vi "myRIO-1900 Quadrotor Sensor FPGA.vi"() -> ()   [LabVIEW 2013]
uses:
  <vilib>/Platform/TimedLoop/XDataNode/timing_clust.ctl
  <vilib>/Platform/TimedLoop/XDataNode/nitl_modes.ctl
  <vilib>/Platform/TimedLoop/XDataNode/wakeup.ctl
  <vilib>/IEDriver/SPIandI2C/FPGA/Private/Initialize Port (I2C).vi
  <vilib>/IEDriver/SPIandI2C/FPGA/Private/IP Port (I2C).vi
  <vilib>/rvi/DataTransferAndStorage/Container/Common/niFpgaContainerGetUniqueNameForEmu.vi
  <vilib>/rvi/DataTransferAndStorage/Container/Common/niFpgaContainerSetEmuInfo.vi
  <vilib>/rvi/eio/common/nirviEmuReportErrorAndStop.vi
  <vilib>/rvi/Emulation/niFpgaSctlEmulationGetInTimedLoop.vi
  <vilib>/rvi/Emulation/niFpgaEmulationReportErrorSimple.vi
  <vilib>/rvi/Emulation/niFpgaGetClockAttributes.vi
  <vilib>/rvi/Emulation/niFpgaCriticalErrorInLSC.vi
  <vilib>/rvi/DataTransferAndStorage/Container/Common/niFpgaContainerExecOnDevCompGetState.vi
  <vilib>/rvi/FIFO/Fifo_Resource/nirvififoEmulationReadFpgaImpl.vi
  <vilib>/rvi/interface/RandomDataEmulation/nirviRandomDataFPGAFIFO.vi
  <vilib>/rvi/interface/RandomDataEmulation/niFpgaRandomDataHandleErrors.vi
  <vilib>/rvi/Memory/Memory_Emulation/nirvimemoryFastEmulationFpgaImpl.vi
  <instcachedir>/0/nirvimemoryFastEmulationFpgaImpl_5FBAB50466BC4C939F684F8805638BFC.lvgen/nirvimemoryFastEmulationFpgaImpl_5FBAB50466BC4C939F684F8805638BFC_005.vi
  <vilib>/rvi/Memory/Memory_Emulation/niFpgaMemoryEmulationCacheClearOnFirstRun.vi
  <vilib>/rvi/Memory/Memory_Emulation/nirvimemoryEmulationManagerCache_MakeExclusive.vi
  <vilib>/rvi/Memory/Memory_Emulation/niFpgaMemoryEmulationValidateCache.vi
  <vilib>/rvi/Memory/Memory_Emulation/nirvimemoryEmulationManagerCache_ReleaseExclusive.vi
  <vilib>/rvi/Memory/Memory_Emulation/nirvimemoryEmulationManagerCache_InsertValue.vi
  <vilib>/Utility/error.llb/Clear Errors.vi
  <vilib>/rvi/Memory/Memory_Emulation/nirvimemoryEmulationManagerCache_GetValue.vi
  <vilib>/rvi/Emulation/niFpgaProcessEmulError.vi
  <vilib>/IEDriver/SPIandI2C/FPGA/Private/Configure Port (I2C).vi
  <vilib>/IEDriver/SPIandI2C/FPGA/Private/Arm Port (I2C).vi
  <vilib>/IEDriver/SPIandI2C/FPGA/Private/Read Port (I2C).vi
  <vilib>/IEDriver/SPIandI2C/FPGA/Private/Write Port (I2C).vi
  <vilib>/rvi/FIFO/Fifo_Resource/nirvififoEmulationWriteFpgaImpl.vi
  <vilib>/rvi/Memory/Memory_Emulation/nirvimemoryEmulationManagerCache_SetValue.vi
  <vilib>/rvi/Emulation/niFpgaSctlEmulationResourceMgr.vi
  <vilib>/Platform/TimedLoop/XDataNode/XDataNode.xnode
  <vilib>/rvi/LocalResourceManager/LocalResourceManager.xnode
  <vilib>/rvi/DataTransferAndStorage/Container/XNode/niFpgaContainer.xnode
  <vilib>/rvi/FIFO/Fifo_Resource/niFpgaFifoEmulationRefIn.vi
  <vilib>/rvi/Memory/Memory_Emulation/niFpgaMemoryEmulationRefIn.vi
  <vilib>/IEDriver/SPIandI2C/FPGA/Library/IP SPI&I2C.lvlib
  <vilib>/Platform/TimedLoop/XDataNode/XDNodeRunTimeDep.lvlib
panel:
  in  "DataAva":bool
  out "GYR_Z":i16
  out "GYR_Y":i16
  out "GYR_X":i16
  out "TEMP":i16
  out "ACC_Z":i16
  out "ACC_Y":i16
  out "ACC_X":i16
  in  "SampleRate_Divider":u32=20000
  in  "WriteData":u8 format="0x%x"
  out "ReadData":u8 format="0x%x"
  in  "CMDParameters":T1
  in  "IICParameters":T2={"Address Type (7-bit)"=enum."7-bit", "IICSlaveAddress"=25, "I2C Parameters"={"Clock Divider"=0}} {"IICSlaveAddress" format="0x%x"}
  in  "ProtocolControl":T3(ring)
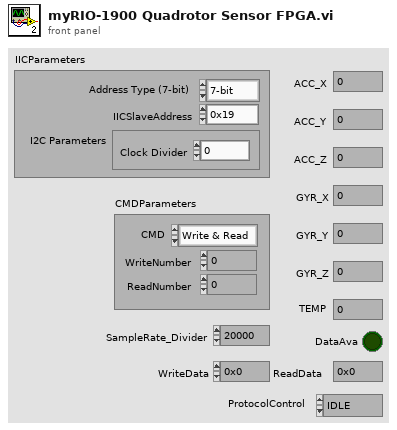
[diagram p1: front panel]
types:
  T1 = cluster{"WriteNumber":u8, "ReadNumber":u8, "CMD":enum8{"Write & Read", "Write", "Read"}}
  T2 = cluster{"Address Type (7-bit)":enum16{"7-bit", "10-bit"}, "IICSlaveAddress":u16, "I2C Parameters":cluster{"Clock Divider":u32}}
  T3 = enum8{"IDLE", "SetIDLE", "Config", "Arm", "Read", "Write", "AutoRead"}
  T4 = cluster{"MPU6050FIFO":refnum<k21>, "MPU6050FIFOAvailable":refnum<k21>}
  T5 = typedef "IP SPI&I2C.lvlib/Private Data (I2C).ctl" = cluster{"Arm Trigger":refnum<k21>, "API to IP Data":refnum<k21>, "IP to API Data":refnum<k21>, "Configuration Register":refnum<k21>, "Configuration Lock":refnum<k21>}
  T6 = typedef "XDNodeRunTimeDep.lvlib/timing_clust.ctl" = cluster{"Expected End [f-1]":u64, "Actual End [f-1]":u64, "Finished Late? [f-1]":bool, "Expected End [i-1]":u64, "Actual End [i-1]":u64, "Finished Late? [i-1]":bool, "Expected Start [i]":u64, "Actual Start [i]":u64, "Expected Start [f]":u64, "Actual Start [f]":u64, "Source Name":string, "Structure Name":string, "Period":i64, "Deadline":i64, "Offset":i64, "Start":i64, "Priority":i32, "Timeout":i32, "Mode":T7, "Wakeup Reason":T8, "Error":errorcluster, "Source Type":string, "Secondary Source Type":string, "Global End Time":u64, "Global Start Time":u64, "Frame Duration":u64, "Iteration Duration":u64, "Assigned CPU":i32, "I/O Scan Engine Mode":u32}
  T7 = typedef "XDNodeRunTimeDep.lvlib/nitl_modes.ctl" = enum32{"No Change", "Process missed periods, maintain original phase", "Discard missed periods, maintain original phase", "Process missed periods, ignore original phase", "Discard missed periods, ignore original phase"}
  T8 = typedef "XDNodeRunTimeDep.lvlib/wakeup.ctl" = enum32{"Normal", "Aborted", "Asynchronous wakeup", "Timing source error", "Timed loop error", "Timeout"}
  T9 = cluster{"NextState":enum16{"Configure", "WriteAddr", "Arm", "Read", "Wait", "Stop"}, "ReadCount":u8, "WaitCounter":u32}
  T10 = enum16{"Configure", "WriteAddr", "Arm", "Read", "Wait", "Stop"}
  T11 = cluster{"NextState":enum8{"IDLE", "ReadData", "Update"}, "ReadCounter":u8, "HighByte":u8}
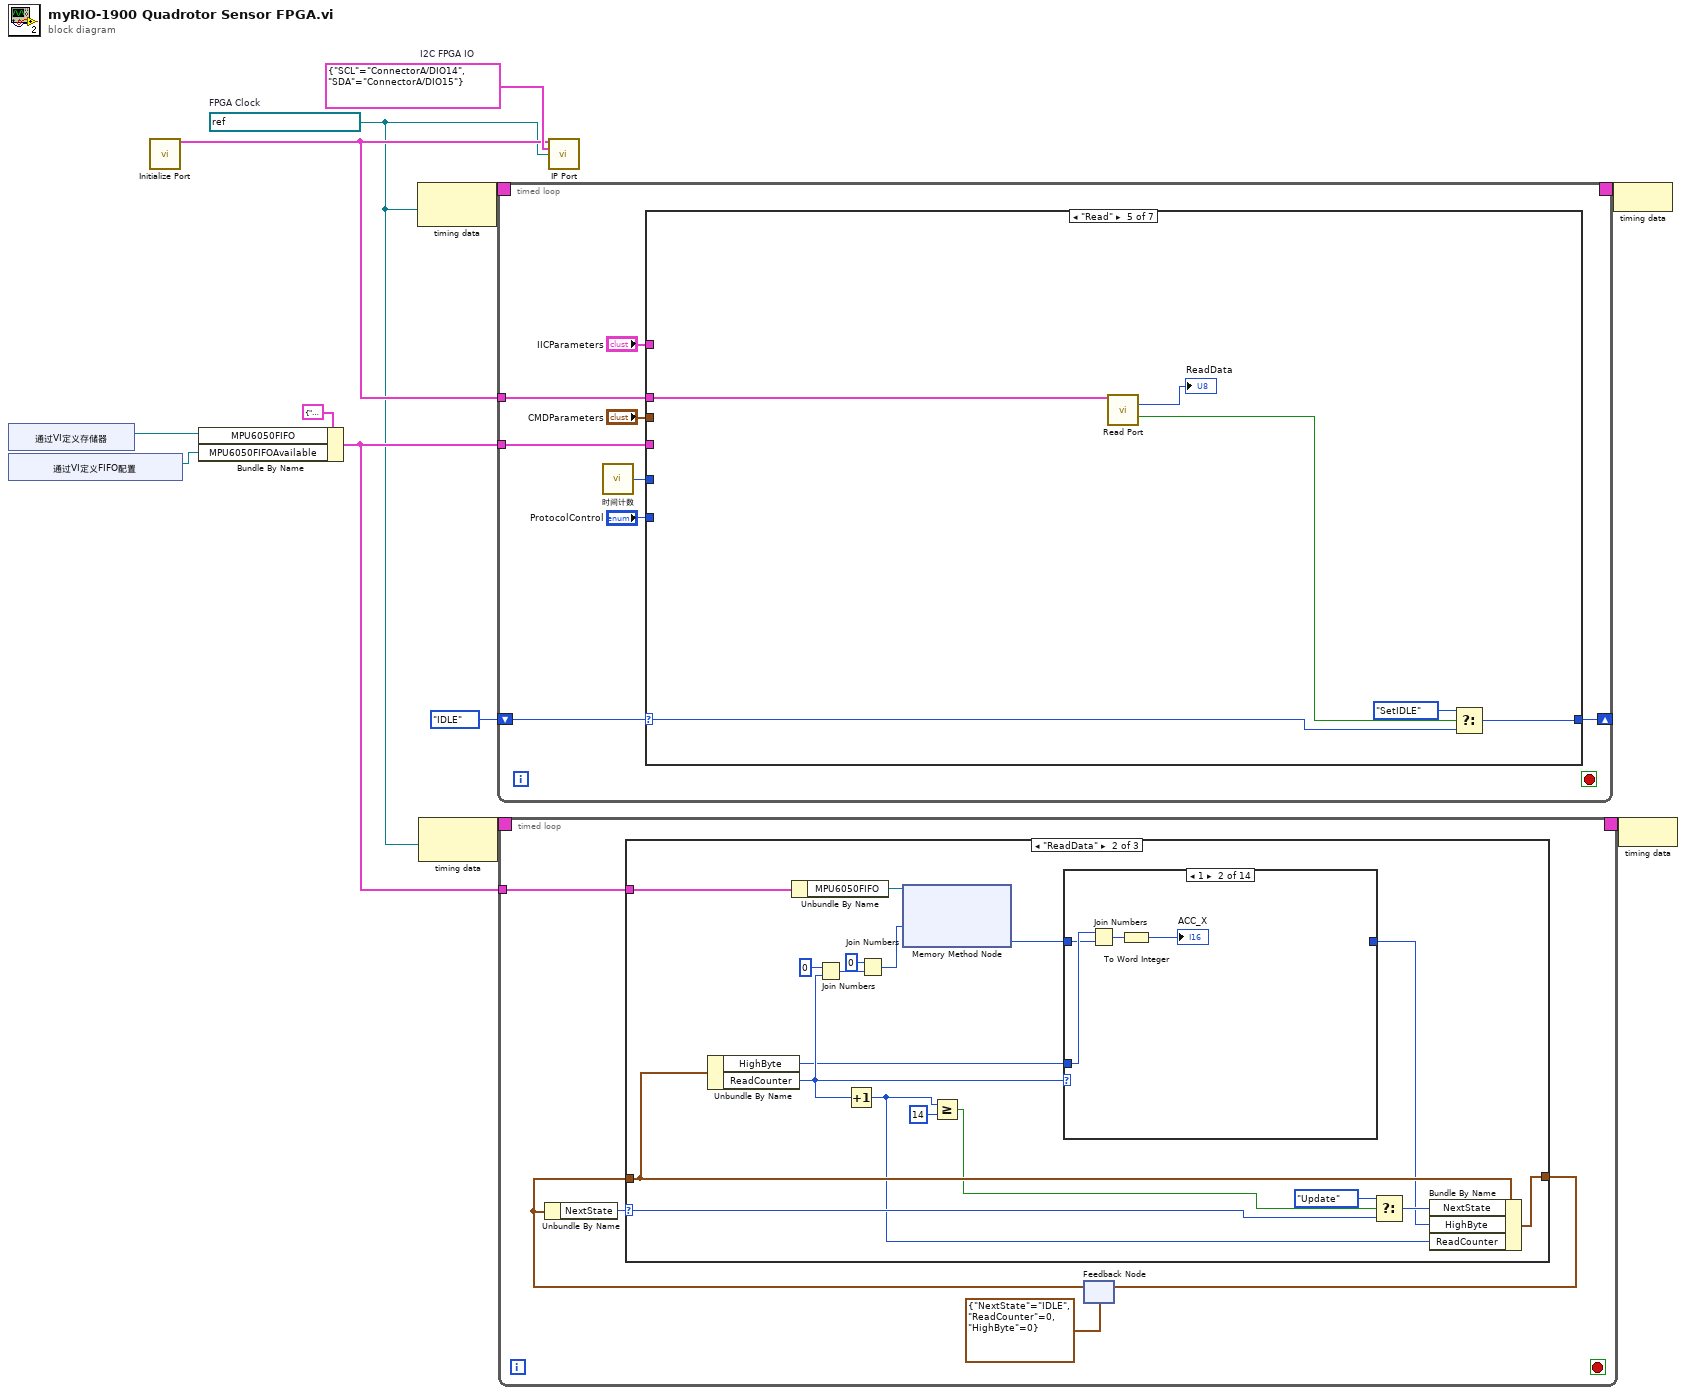
[diagram p0: block diagram]
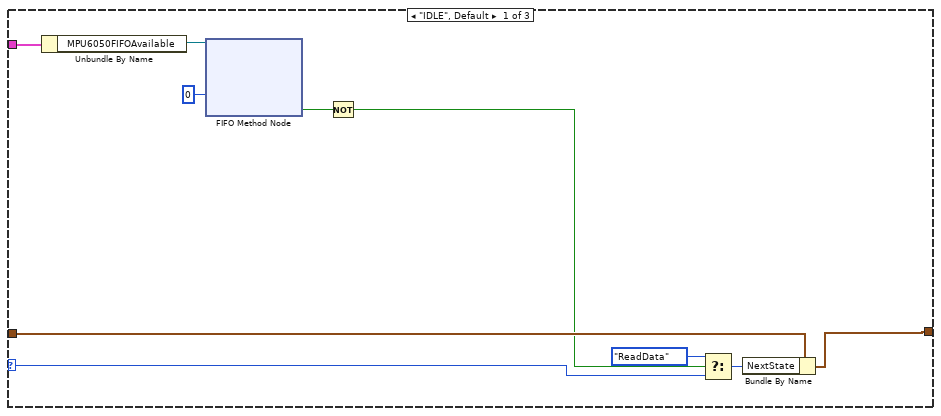
[diagram p2: hidden frame]
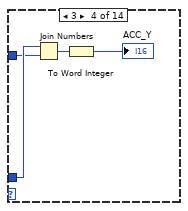
[diagram p5: hidden frame]
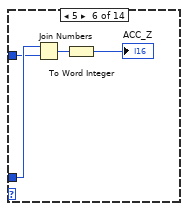
[diagram p7: hidden frame]
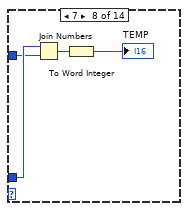
[diagram p9: hidden frame]
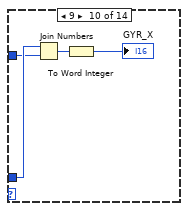
[diagram p11: hidden frame]
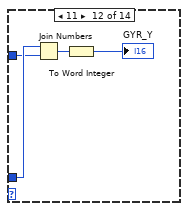
[diagram p13: hidden frame]
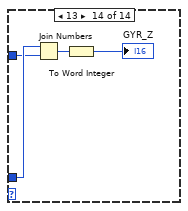
[diagram p15: hidden frame]
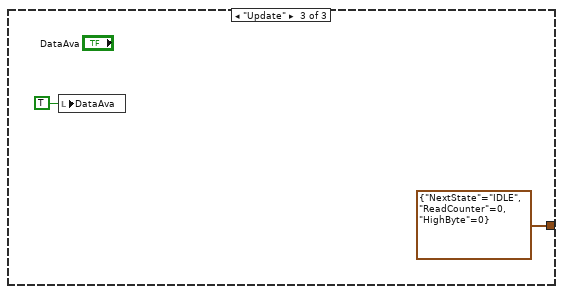
[diagram p16: hidden frame]
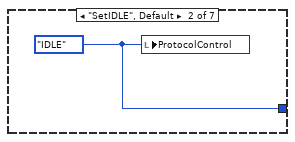
[diagram p18: hidden frame]
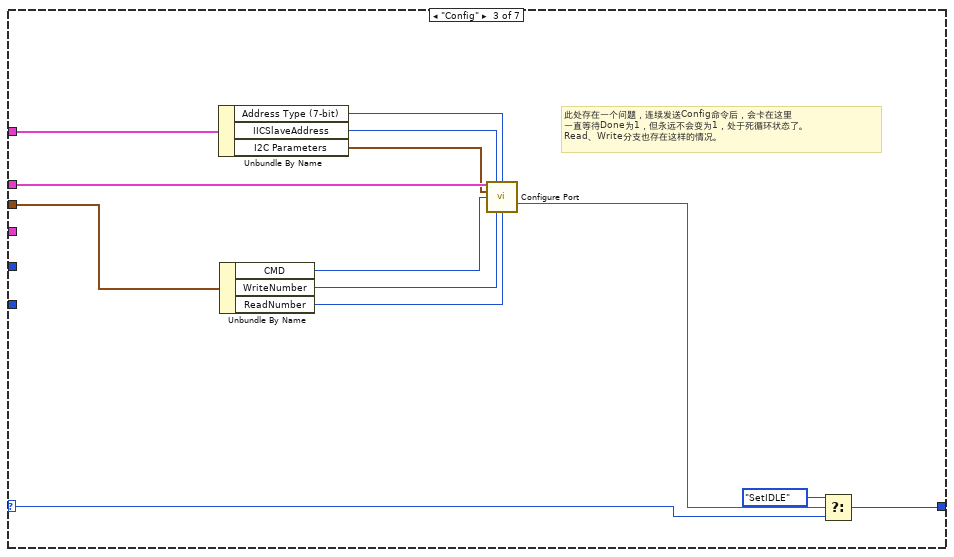
[diagram p19: hidden frame]
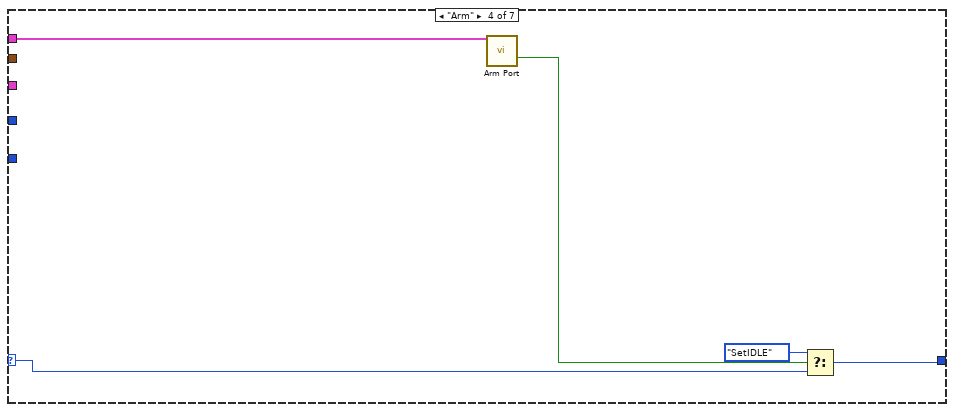
[diagram p20: hidden frame]
diagram:
  w1 = refnum<k21> "40 MHz Onboard Clock"  # FPGA Clock
  w8 = cluster{"SCL":refnum<k21>, "SDA":refnum<k21>} {"SCL"="ConnectorA/DIO14", "SDA"="ConnectorA/DIO15"}  # I2C FPGA IO
  n1 = xnode "通过VI定义存储器"() -> ("存储器输出"=w4:refnum<k21>)
  n2 = xnode "通过VI定义FIFO配置"() -> ("FIFO输出"=w3:refnum<k21>)
  n3 = call-poly <vilib>:"Initialize Port.vi"() -> ("Private Data Out"=w7:T5)  [unwired: 14 in, 1 out]
  n4 = Bundle By Name(cluster=T4 {"MPU6050FIFO"="", "MPU6050FIFOAvailable"=""}, "MPU6050FIFO"=w4, "MPU6050FIFOAvailable"=w3) -> (w2:T4)
  n5 = node-c288(w1) -> (w12:T6)
  n6 = node-c288(w1) -> (w10:T6)
  n7 = timed-loop {
    tunnel: w7 -> [w18]
    shift-right: [w15] -> _
    shift-left: T3."IDLE" ("ProtocolControl") -> [w20]
    timing: w12 -> [_]
    timing-out: [_] -> w11
    tunnel: w2 -> [w13]
    stop <- _ stop-if-true
    n8 = call "时间计数"() -> ("Tick Count(Ticks)"=w14:u32)
    n9 = case shown="\"Read\"" w20 {
      selector: w20 -> [_ _ w35 w38 w45 w50 w63]
      tunnel: "CMDParameters" -> [_ _ w28 _ _ _ _]
      tunnel: w18 -> [_ _ w34 w40 w46 w52 w59]
      tunnel: "IICParameters" -> [_ _ w32 _ _ _ w58]
      tunnel: "ProtocolControl" -> [w21 _ _ _ _ _ w57]
      tunnel: [w21 w22 w24 w37 w42 w48 w64] -> w15
      tunnel: w14 -> [_ _ _ _ _ _ w55]
      tunnel: w13 -> [_ _ _ _ _ _ w54]
      frame "IDLE" {
      }
      frame "SetIDLE", Default {
        w22 = T3."IDLE" ("ProtocolControl")
        n10 = local write "ProtocolControl"(w22) -> ()
      }
      frame "Config" {
        # "此处存在一个问题，连续发送Config命令后，会卡在这里\n一直等待Done为1，但永远不会变为1，处于死循环状态了。\nRead、Write分支也存在这样的情况。"
        n11 = Unbundle By Name(w32) -> ("Address Type (7-bit)"=w31:enum16{"7-bit", "10-bit"}, "IICSlaveAddress"=w30:u16, "I2C Parameters"=w29:cluster{"Clock Divider":u32})
        n12 = Unbundle By Name(w28) -> ("CMD"=w27:enum8{"Write & Read", "Write", "Read"}, "WriteNumber"=w26:u8, "ReadNumber"=w25:u8)
        n13 = call-poly <vilib>:"Configure Port.vi"("Private Data In"=w34, "Address"=w30, "Address Type (7-bit)"=w31, "I2C Parameters"=w29, "Command (Write & Read)"=w27, "Number of Bytes to Write"=w26, "Number of Bytes to Read"=w25) -> ("Done"=w33:bool)  [unwired: 6 in, 2 out]
        n14 = Select(t=T3."SetIDLE", s=w33, f=w35) -> (s? t:f=w24:T3)
      }
      frame "Arm" {
        n15 = call-poly <vilib>:"Arm Port.vi"("Private Data In"=w40) -> ("Done"=w39:bool)  [unwired: 12 in, 2 out]
        n16 = Select(t=T3."SetIDLE", s=w39, f=w38) -> (s? t:f=w37:T3)
      }
      frame "Read" {
        n17 = call-poly <vilib>:"Read Port.vi"("Private Data In"=w46) -> ("Data Out"=→"ReadData":u8, "Output Valid"=w44:bool)  [unwired: 11 in, 2 out]
        n18 = Select(t=T3."SetIDLE", s=w44, f=w45) -> (s? t:f=w42:T3)
      }
      frame "Write" {
        n19 = call-poly <vilib>:"Write Port.vi"("Private Data In"=w52, "Data In"="WriteData") -> ("Done"=w49:bool)  [unwired: 11 in, 2 out]
        n20 = Select(t=T3."SetIDLE", s=w49, f=w50) -> (s? t:f=w48:T3)
      }
      frame "AutoRead" {
        n21 = feedback #1(T9 {"NextState"=enum."Configure", "ReadCount"=0, "WaitCounter"=0}) -> (w61:T9)
        n22 = Unbundle By Name(w61) -> ("NextState"=w53:T10)
        n23 = case shown="\"Read\"" w53 {
          selector: w53 -> [w70 w84 w93 w104 w129 _]
          tunnel: w61 -> [w72 w83 w91 w102 w131 _]
          tunnel: [w71 w82 w92 w103 w130 T9 {"NextState"=enum."Configure", "ReadCount"=0, "WaitCounter"=0}] -> w60
          tunnel: w59 -> [w80 w88 w90 w107 _ _]
          tunnel: w58 -> [w79 _ _ _ _ _]
          tunnel: w57 -> [_ _ _ _ _ w137]
          tunnel: [_ _ _ _ _ w135] -> w56
          tunnel: w55 -> [w66 _ _ _ w125 _]
          tunnel: w54 -> [_ _ _ w97 _ _]
          frame "Configure", Default {
            w75 = u8 0 items=["Write & Read", "Write", "Read"] ("Command (Write & Read)")
            # "NO Done"
            n24 = Unbundle By Name(w79) -> ("Address Type (7-bit)"=w78:enum16{"7-bit", "10-bit"}, "IICSlaveAddress"=w77:u16, "I2C Parameters"=w76:cluster{"Clock Divider":u32})
            n25 = call-poly <vilib>:"Configure Port.vi"("Private Data In"=w80, "Address"=w77, "Address Type (7-bit)"=w78, "I2C Parameters"=w76, "Command (Write & Read)"=w75, "Number of Bytes to Write"=u16 1, "Number of Bytes to Read"=u16 14) -> ("Done"=w68:bool)  [unwired: 6 in, 2 out]
            n26 = Select(t=T10."WriteAddr", s=w68, f=w70) -> (s? t:f=w69:T10)
            n27 = Bundle By Name(cluster=w72, "NextState"=w69, "WaitCounter"=w66) -> (w71:T9)
          }
          frame "WriteAddr" {
            n28 = call-poly <vilib>:"Write Port.vi"("Private Data In"=w88, "Data In"=u8 59) -> ("Done"=w81:bool)  [unwired: 11 in, 2 out]
            n29 = Select(t=T10."Arm", s=w81, f=w84) -> (s? t:f=w86:T10)
            n30 = Bundle By Name(cluster=w83, "NextState"=w86) -> (w82:T9)
          }
          frame "Arm" {
            n31 = call-poly <vilib>:"Arm Port.vi"("Private Data In"=w90) -> ("Done"=w89:bool)  [unwired: 12 in, 2 out]
            n32 = Select(t=T10."Read", s=w89, f=w93) -> (s? t:f=w95:T10)
            n33 = Bundle By Name(cluster=w91, "NextState"=w95) -> (w92:T9)
          }
          frame "Read" {
            n34 = Unbundle By Name(w102) -> ("ReadCount"=w106:u8)
            n35 = call-poly <vilib>:"Read Port.vi"("Private Data In"=w107) -> ("Data Out"=w105:u8, "Output Valid"=w96:bool)  [unwired: 11 in, 2 out]
            n36 = case shown="假" w96 {
              tunnel: w106 -> [w111 w120]
              tunnel: w105 -> [_ w117]
              tunnel: [w111 w124] -> w100
              tunnel: w97 -> [w112 w119]
              frame False {
                n37 = Unbundle By Name(w112) -> ("MPU6050FIFOAvailable"=w109:refnum<k21>)
                n38 = Less Or Equal?(x=u8 13, y=w111) -> (x <= y?=w108:bool)
                n39 = case shown="真" w108 {
                  tunnel: w109 -> [_ w115]
                  frame False {
                  }
                  frame True {
                    n40 = xnode ("FIFO Method Node")("元素"=TRUE, "超时"=0, "FIFO输入"=w115) -> ()  [unwired: 2 out]
                  }
                }
              }
              frame True {
                n41 = Unbundle By Name(w119) -> ("MPU6050FIFO"=w118:refnum<k21>)
                n42 = Join Numbers(hi=u8 0, lo=w120) -> ((hi.lo)=w123:u16)
                n43 = Join Numbers(hi=u16 0, lo=w123) -> ((hi.lo)=w116:u32)
                n44 = Increment(x=w120) -> (x+1=w124:u8)
                n45 = xnode ("Memory Method Node")("地址"=w116, "数据"=w117, "存储器输入"=w118) -> ()  [unwired: 1 out]
              }
            }
            n46 = Not(x=w96) -> (.not. x?=w99:bool)
            n47 = Select(t=T10."Wait", s=w99, f=w104) -> (s? t:f=w101:T10)
            n48 = Bundle By Name(cluster=w102, "ReadCount"=w100, "NextState"=w101) -> (w103:T9)
          }
          frame "Wait" {
            n49 = Unbundle By Name(w131) -> ("WaitCounter"=w134:u32)
            n50 = Subtract(x=w125, y=w134) -> (x-y=w133:u32)
            n51 = Less?(x="SampleRate_Divider", y=w133) -> (x < y?=w127:bool)
            n52 = Select(t=T10."Stop", s=w127, f=w129) -> (s? t:f=w128:T10)
            n53 = Bundle By Name(cluster=w131, "NextState"=w128) -> (w130:T9)
          }
          frame "Stop" {
            # "Done"
            n54 = Equal?(x=T3."SetIDLE", y=w137) -> (x = y?=w135:bool)
          }
        }
        n55 = feedback-in #1(w60) -> ()
        n56 = Select(t=T3."SetIDLE", s=w56, f=w63) -> (s? t:f=w64:T3)
      }
    }
  }
  n57 = timed-loop {
    tunnel: w2 -> [w142]
    timing: w10 -> [_]
    timing-out: [_] -> w9
    stop <- _ stop-if-true
    n58 = feedback #2(T11 {"NextState"=enum."IDLE", "ReadCounter"=0, "HighByte"=0}) -> (w144:T11)
    n59 = Unbundle By Name(w144) -> ("NextState"=w143:enum8{"IDLE", "ReadData", "Update"})
    n60 = case shown="\"ReadData\"" w143 {
      selector: w143 -> [w150 w164 _]
      tunnel: w144 -> [w152 w166 _]
      tunnel: w142 -> [w155 w173 _]
      tunnel: [w151 w165 T11 {"NextState"=enum."IDLE", "ReadCounter"=0, "HighByte"=0}] -> w141
      frame "IDLE", Default {
        n61 = Unbundle By Name(w155) -> ("MPU6050FIFOAvailable"=w154:refnum<k21>)
        n62 = xnode ("FIFO Method Node")("超时"=0, "FIFO输入"=w154) -> ("超时？"=w148:bool)  [unwired: 2 out]
        n63 = Not(x=w148) -> (.not. x?=w147:bool)
        n64 = Select(t=enum8{"IDLE", "ReadData", "Update"}."ReadData", s=w147, f=w150) -> (s? t:f=w149:enum8{"IDLE", "ReadData", "Update"})
        n65 = Bundle By Name(cluster=w152, "NextState"=w149) -> (w151:T11)
      }
      frame "ReadData" {
        n66 = Unbundle By Name(w166) -> ("HighByte"=w157:u8, "ReadCounter"=w160:u8)
        n67 = Unbundle By Name(w173) -> ("MPU6050FIFO"=w172:refnum<k21>)
        n68 = Join Numbers(hi=u8 0, lo=w160) -> ((hi.lo)=w171:u16)
        n69 = Increment(x=w160) -> (x+1=w156:u8)
        n70 = Join Numbers(hi=u16 0, lo=w171) -> ((hi.lo)=w168:u32)
        n71 = xnode ("Memory Method Node")("地址"=w168, "存储器输入"=w172) -> ("数据"=w159:u8)  [unwired: 1 out]
        n72 = Greater Or Equal?(x=w156, y=u8 14) -> (x >= y?=w162:bool)
        n73 = case shown="1" w160 {
          tunnel: w159 -> [w174 w177 w179 w182 w184 w187 w189 w192 w194 w197 w199 w202 w204 w207]
          tunnel: [w174 _ w179 _ w184 _ w189 _ w194 _ w199 _ w204 _] -> w158
          tunnel: w157 -> [_ w178 _ w183 _ w188 _ w193 _ w198 _ w203 _ w208]
          frame 0, Default {
          }
          frame 1 {
            n74 = Join Numbers(hi=w178, lo=w177) -> ((hi.lo)=w176:u16)
            n75 = To Word Integer(number=w176) -> (16bit integer=→"ACC_X":i16)
          }
          frame 2 {
          }
          frame 3 {
            n76 = Join Numbers(hi=w183, lo=w182) -> ((hi.lo)=w181:u16)
            n77 = To Word Integer(number=w181) -> (16bit integer=→"ACC_Y":i16)
          }
          frame 4 {
          }
          frame 5 {
            n78 = Join Numbers(hi=w188, lo=w187) -> ((hi.lo)=w186:u16)
            n79 = To Word Integer(number=w186) -> (16bit integer=→"ACC_Z":i16)
          }
          frame 6 {
          }
          frame 7 {
            n80 = Join Numbers(hi=w193, lo=w192) -> ((hi.lo)=w191:u16)
            n81 = To Word Integer(number=w191) -> (16bit integer=→"TEMP":i16)
          }
          frame 8 {
          }
          frame 9 {
            n82 = Join Numbers(hi=w198, lo=w197) -> ((hi.lo)=w196:u16)
            n83 = To Word Integer(number=w196) -> (16bit integer=→"GYR_X":i16)
          }
          frame 10 {
          }
          frame 11 {
            n84 = Join Numbers(hi=w203, lo=w202) -> ((hi.lo)=w201:u16)
            n85 = To Word Integer(number=w201) -> (16bit integer=→"GYR_Y":i16)
          }
          frame 12 {
          }
          frame 13 {
            n86 = Join Numbers(hi=w208, lo=w207) -> ((hi.lo)=w206:u16)
            n87 = To Word Integer(number=w206) -> (16bit integer=→"GYR_Z":i16)
          }
        }
        n88 = Select(t=enum8{"IDLE", "ReadData", "Update"}."Update", s=w162, f=w164) -> (s? t:f=w163:enum8{"IDLE", "ReadData", "Update"})
        n89 = Bundle By Name(cluster=w166, "NextState"=w163, "HighByte"=w158, "ReadCounter"=w156) -> (w165:T11)
      }
      frame "Update" {
        n90 = local write "DataAva"(TRUE ("DataAva")) -> ()
      }
    }
    n91 = feedback-in #2(w141) -> ()
  }
  n92 = call-poly <vilib>:"IP Port.vi"("Private Data In"=w7, "I2C FPGA IO"=w8, "FPGA Clock"=w1) -> ()  [unwired: 13 in]
  n93 = node-c288(w11) -> ()
  n94 = node-c288(w9) -> ()
